vi "PV Handheld Change logging value.vi"(10 "response logging data in":string) -> (0 "end of logging value":bool, 1 "Intervaltime out (s)":string, 2 "Pressure out":string, 3 "logging Array out":string[](array[string]))   [LabVIEW 2016, in "Pfeiffer Vacuum.lvlib"]
uses:
  Pfeiffer Vacuum.lvlib
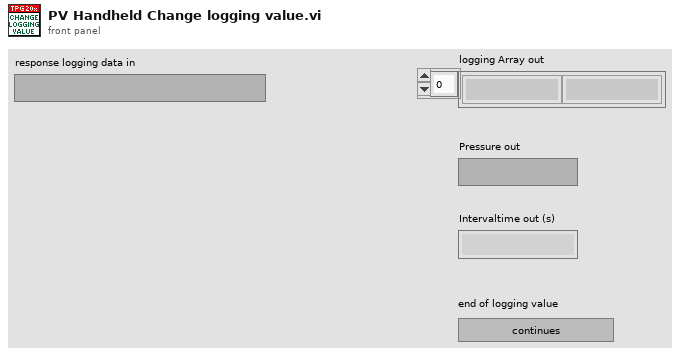
[diagram p1: front panel]
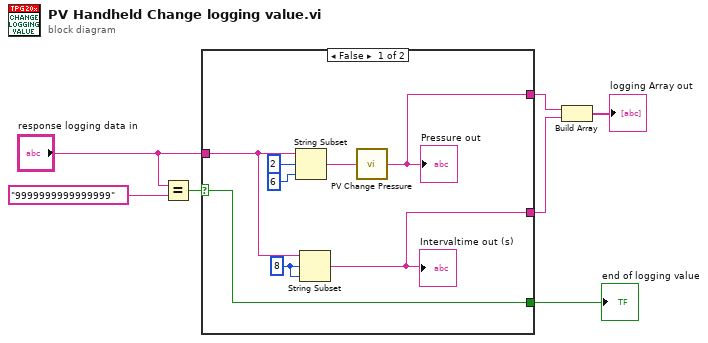
[diagram p0: block diagram]
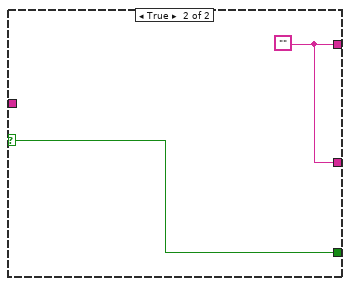
[diagram p2: hidden frame]
diagram:
  n1 = Equal?(x="response logging data in", y="9999999999999999" ("Maximalwert")) -> (x = y?=w7:bool)
  n2 = case shown="False" w7 {
    selector: w7 -> [w8 w16]
    tunnel: "response logging data in" -> [w11 _]
    tunnel: [w10 w17] -> w4
    tunnel: [w9 w17] -> w3
    tunnel: [w8 w16] -> w1
    frame False {
      w13 = 8 ("Offset (0)")
      n3 = String Subset(string=w11, offset (0)=2 ("Offset (0)"), length (rest)=6 ("Offset (0)")) -> (substring=w12:string)
      n4 = String Subset(string=w11, offset (0)=w13, length (rest)=w13) -> (substring=w9:string)
      "Intervaltime out (s)" <- w9
      n5 = call "PV Change Pressure.vi"("Pressure String"=w12) -> ("Change Pressure String"=w10:string)
      "Pressure out" <- w10
    }
    frame True {
      w17 = ""
    }
  }
  "end of logging value" <- w1
  n6 = Build Array(w4, w3) -> (→"logging Array out":string[])
